vi "CSDB_Config.insert data.vi"(1 "InstanceID":string, 2 "AttributeID":string, 3 "Value":string, 5 "error in (no error)":errorcluster) -> (19 "error out":errorcluster)   [LabVIEW 2014, in "CSDB_Config.lvlib"]
doc: "write data of an attribute element to the data base"
uses:
  CSDB_Config.lvlib
  <vilib>/addons/database/NI_Database_API.lvlib
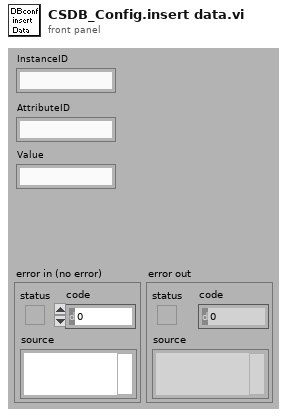
[diagram p1: front panel]
types:
  T1 = typedef "NI_Database_API.lvlib/Conn ObjectReference.ctl" = refnum<k1>
  T2 = cluster{"InstanceID":string, "AttributeID":string, "Value":string}
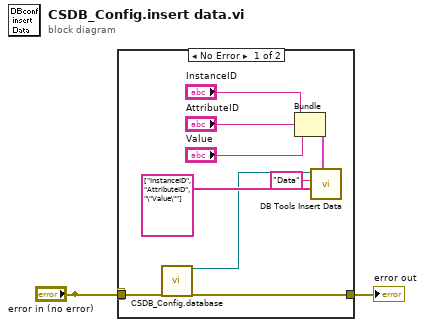
[diagram p0: block diagram]
diagram:
  n1 = case shown="No Error" "error in (no error)" {
    selector: "error in (no error)" -> [_ w12]
    tunnel: "error in (no error)" -> [w5 _]
    tunnel: [w4 w12] -> w2
    frame No Error {
      n2 = call "CSDB_Config.database.vi"("error in (no error)"=w5) -> ("connectionRef out"=w3:T1, "error out"=w4:errorcluster)  [unwired: 17 in]
      n3 = Bundle("InstanceID"="InstanceID", "AttributeID"="AttributeID", "Value"="Value") -> (w7:T2)  [unwired: 1 in]
      n4 = call <vilib>:"DB Tools Insert Data.vi"("data"=w7, "columns"=string[] ["InstanceID", "AttributeID", "\"Value\""], "table"="Data", "connection reference"=w3) -> ()  [unwired: 6 in, 2 out]
    }
    frame Error {
    }
  }
  "error out" <- w2
